vi "ArdnoManualControl.vi"() -> ()   [LabVIEW 2018, in "Arduino.lvlib"]
uses:
  Arduino.lvlib
  <vilib>/MakerHub/LINX/Public/Peripherals/Digital/Digital Write N Chans.vi
  <vilib>/MakerHub/LINX/Private/Local IO/LinxDigitalWrite.vi
  <vilib>/MakerHub/LINX/Public/Utilities/Check Channel.vi
  <vilib>/MakerHub/LINX/Public/Utilities/Open Serial.vi
  <vilib>/MakerHub/LINX/Private/Utilties/Generate Error.vi
  <vilib>/MakerHub/LINX/LMH-LINX.lvlib
panel:
  in  "Valve (A1-C8),\n comma separated":string
  in  "stop":bool
  in  "Change State\n (XOR)":bool
  in  "Period on (=Period off) (ms)":i32
  in  "All close":bool=TRUE
  in  "All open":bool
  in  "Valve (A1-C8),\n comma separated 2":string
  in  "Valve Port (Arduino)":refnum<visa-resource-name>="COM7"
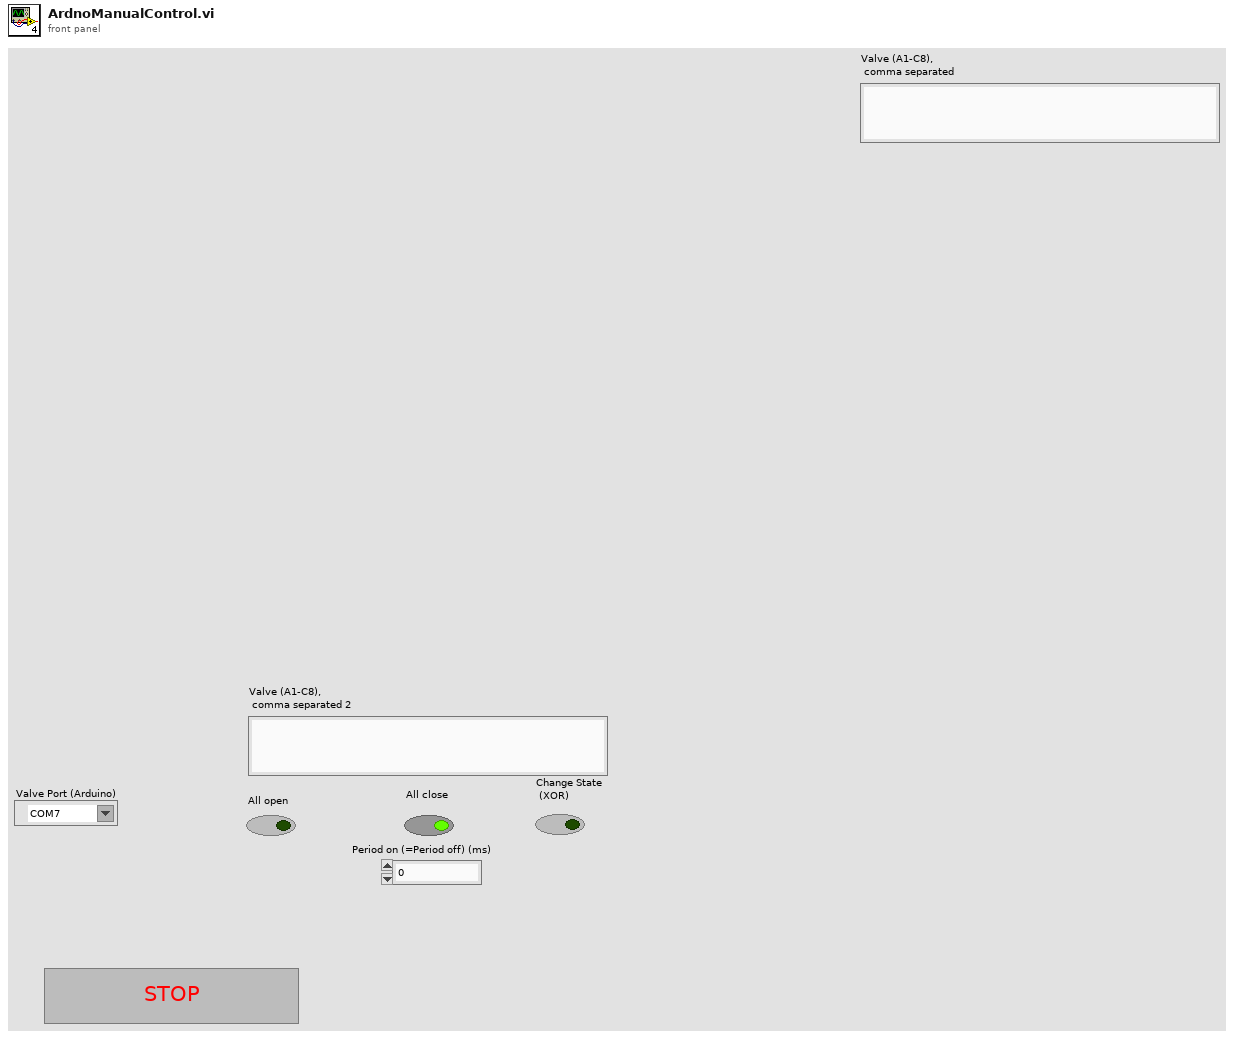
[diagram p1: front panel]
types:
  T1 = typedef "LMH-LINX.lvlib/LINX Ref.ctl" = cluster{"IO":T2, "Interface":T3, "LINX Device Config":T4}
  T2 = typedef "LMH-LINX.lvlib/Platform.ctl" = enum16{"Remote", "Local"}
  T3 = typedef "LMH-LINX.lvlib/Interface.ctl" = enum16{"Serial", "TCP"}
  T4 = typedef "LMH-LINX.lvlib/Device.lvlib/LINX Device Config.ctl" = cluster{"Interface":T3, "COM Port":refnum<visa-resource-name>, "TCP Configuration":T5, "Device Family":u8, "Device ID":u8, "Device Name":string, "TCP Ref":refnum<k5>, "Channels":T6}
  T5 = typedef "LMH-LINX.lvlib/Device.lvlib/TCP Config.ctl" = cluster{"IP Address":string, "Port":u16}
  T6 = typedef "LMH-LINX.lvlib/Channels.ctl" = cluster{"DI":u8[], "DO":u8[], "AI":u8[], "AO":u8[], "PWM":u8[], "QE":u8[], "UART":u8[], "I2C 2":u8[], "SPI":u8[], "CAN":u8[], "Servo":u8[], "AI Ref (V)":dbl, "AI Resolution (Bits)":u8, "AO Ref (V)":dbl, "AO Resolution (Bits)":u8}
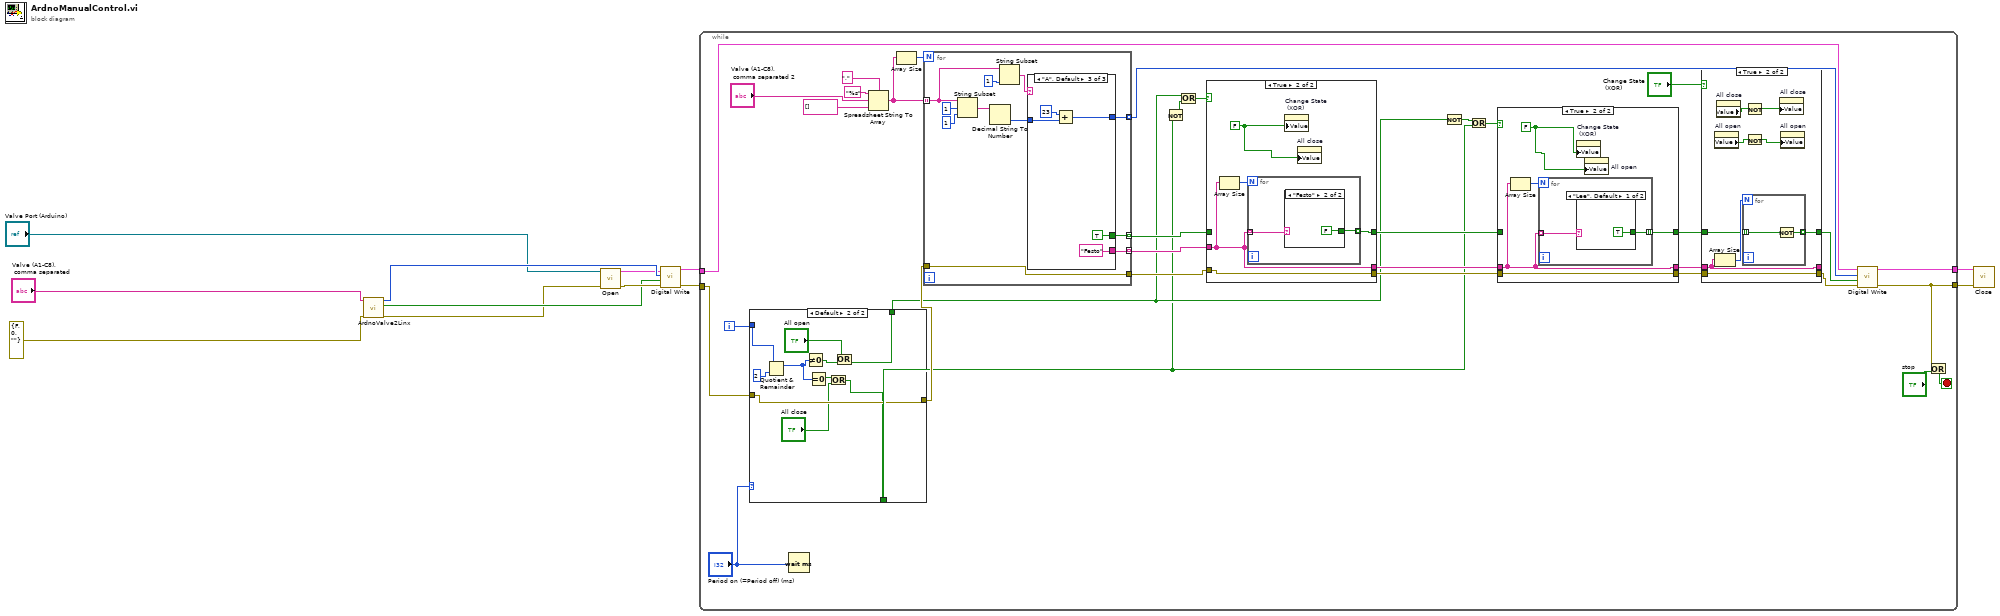
[diagram p0: block diagram]
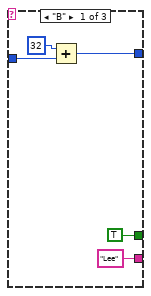
[diagram p2: hidden frame]
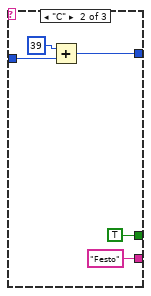
[diagram p3: hidden frame]
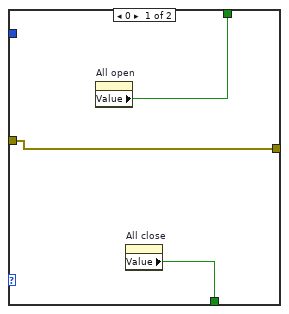
[diagram p4: hidden frame]
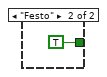
[diagram p7: hidden frame]
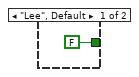
[diagram p9: hidden frame]
diagram:
  n1 = call "ArdnoValve2Linx.vi"("error in (no error)"=errorcluster {"status"=FALSE, "code"=0, "source"=""}, "Valve (A1-C8),\n comma separated"="Valve (A1-C8),\n comma separated") -> ("error out"=w5:errorcluster, "Closed State"=w6:bool[], "Linx Port"=w7:i32[])  [unwired: 7 in]
  n2 = call-poly <vilib>:"Open.vi"("Error In"=w5, "Serial Port"="Valve Port (Arduino)") -> ("Error Out"=w10:errorcluster, "LINX Resource"=w1:T1)  [unwired: 7 in, 1 out]
  n3 = call-poly <vilib>:"Digital Write.vi"("Error In"=w10, "Values"=w6, "DO Channels"=w7, "LINX Resource"=w1) -> ("Error Out"=w9:errorcluster, "LINX Resource"=w8:T1)  [unwired: 6 in]
  n4 = while {
    tunnel: w8 -> [w37]
    tunnel: w9 -> [w26]
    tunnel: [w35] -> w11
    tunnel: [w36] -> w12
    i -> [w28]
    stop <- w34 stop-if-true
    n5 = case shown="Default" "Period on (=Period off) (ms)" {
      tunnel: w28 -> [_ w85]
      tunnel: w26 -> [w75 w82]
      tunnel: [w75 w82] -> w24
      tunnel: [w74 w77] -> w20
      tunnel: [w73 w80] -> w19
      frame 0 {
        n6 = property on="All open" class="Bool (strict)"() -> ("Value"=w74:bool)  [unwired: 2 in, 2 out]
        n7 = property on="All close" class="Bool (strict)"() -> ("Value"=w73:bool)  [unwired: 2 in, 2 out]
      }
      frame Default {
        n8 = Quotient & Remainder(x=w85, y=2) -> (x-y*floor(x/y)=w83:i32)  [unwired: 1 out]
        n9 = Not Equal To 0?(x=w83) -> (x != 0?=w81:bool)
        n10 = Equal To 0?(x=w83) -> (x = 0?=w79:bool)
        n11 = Or(x=w79, y="All close") -> (x .or. y?=w80:bool)
        n12 = Or(x="All open", y=w81) -> (x .or. y?=w77:bool)
      }
    }
    n13 = Wait (ms)(milliseconds to wait="Period on (=Period off) (ms)") -> ()  [unwired: 1 out]
    n14 = Spreadsheet String To Array(delimiter (Tab)=",", format string="%s", spreadsheet string="Valve (A1-C8),\n comma separated 2", array type (2D Dbl)=string[] []) -> (array=w18:string[])
    n15 = Array Size(array=w18) -> (size(s)=w17:i32)
    n16 = for {
      N: w17 -> [_]
      tunnel: w18 -> [w54] mode=indexing
      tunnel: [w49] -> w45 mode=indexing
      tunnel: [w50] -> w46 mode=indexing
      tunnel: [w48] -> w38 mode=indexing
      tunnel: [w47] -> w25
      tunnel: w24 -> [w47]
      n17 = String Subset(string=w54, offset (0)=1, length (rest)=1 ("length (rest)")) -> (substring=w52:string)
      n18 = Decimal String To Number(string=w52) -> (number=w51:i32)  [unwired: 2 in, 1 out]
      n19 = String Subset(string=w54, length (rest)=1 ("length (rest)")) -> (substring=w56:string)  [unwired: 1 in]
      n20 = case shown="\"A\", Default" w56 {
        tunnel: [w61 w66 w71] -> w48
        tunnel: w51 -> [w60 w65 w70]
        tunnel: ["Lee" "Festo" "Festo"] -> w50
        tunnel: [TRUE TRUE TRUE] -> w49
        frame "B" {
          n21 = Add(x=32, y=w60) -> (x+y=w61:i32)
        }
        frame "C" {
          n22 = Add(x=39, y=w65) -> (x+y=w66:i32)
        }
        frame "A", Default {
          n23 = Add(x=23, y=w70) -> (x+y=w71:i32)
        }
      }
    }
    n24 = Not(x=w19) -> (.not. x?=w29:bool)
    n25 = Or(x=w20, y=w29) -> (x .or. y?=w30:bool)
    n26 = case shown="True" w30 {
      tunnel: w46 -> [w110 w114]
      tunnel: w45 -> [w111 _]
      tunnel: [w111 w115] -> w44
      tunnel: [w110 w114] -> w43
      tunnel: w25 -> [_ w112]
      tunnel: [_ w112] -> w23
      frame False {
      }
      frame True {
        w113 = FALSE
        n27 = Array Size(array=w114) -> (size(s)=w116:i32)
        n28 = for {
          N: w116 -> [_]
          tunnel: w114 -> [w118] mode=indexing
          tunnel: [w117] -> w115 mode=indexing
          n29 = case shown="\"Festo\"" w118 {
            tunnel: [FALSE FALSE] -> w117
            frame "Lee", Default {
            }
            frame "Festo" {
            }
          }
        }
        n30 = property on="Change State\n (XOR)" class="Bool (strict)"("Value"=w113) -> ()  [unwired: 2 in, 2 out]
        n31 = property on="All close" class="Bool (strict)"("Value"=w113) -> ()  [unwired: 2 in, 2 out]
      }
    }
    n32 = Not(x=w20) -> (.not. x?=w31:bool)
    n33 = Or(x=w31, y=w19) -> (x .or. y?=w32:bool)
    n34 = case shown="True" w32 {
      tunnel: w43 -> [w99 w103]
      tunnel: w44 -> [w100 _]
      tunnel: [w100 w104] -> w41
      tunnel: [w99 w103] -> w40
      tunnel: w23 -> [_ w101]
      tunnel: [_ w101] -> w22
      frame False {
      }
      frame True {
        w102 = FALSE
        n35 = Array Size(array=w103) -> (size(s)=w105:i32)
        n36 = for {
          N: w105 -> [_]
          tunnel: w103 -> [w107] mode=indexing
          tunnel: [w106] -> w104 mode=indexing
          n37 = case shown="\"Lee\", Default" w107 {
            tunnel: [TRUE TRUE] -> w106
            frame "Lee", Default {
            }
            frame "Festo" {
            }
          }
        }
        n38 = property on="Change State\n (XOR)" class="Bool (strict)"("Value"=w102) -> ()  [unwired: 2 in, 2 out]
        n39 = property on="All open" class="Bool (strict)"("Value"=w102) -> ()  [unwired: 2 in, 2 out]
      }
    }
    n40 = case shown="True" "Change State\n (XOR)" {
      tunnel: w40 -> [w86 w94]
      tunnel: w41 -> [w87 w93]
      tunnel: [w87 w95] -> w39
      tunnel: [w86 w94] -> _
      tunnel: w22 -> [_ w92]
      tunnel: [_ w92] -> w21
      frame False {
      }
      frame True {
        n41 = property on="All open" class="Bool (strict)"() -> ("Value"=w88:bool)  [unwired: 2 in, 2 out]
        n42 = Array Size(array=w94) -> (size(s)=w96:i32)
        n43 = property on="All close" class="Bool (strict)"() -> ("Value"=w91:bool)  [unwired: 2 in, 2 out]
        n44 = for {
          N: w96 -> [_]
          tunnel: [w97] -> w95 mode=indexing
          tunnel: w93 -> [w98] mode=indexing
          n45 = Not(x=w98) -> (.not. x?=w97:bool)
        }
        n46 = Not(x=w91) -> (.not. x?=w90:bool)
        n47 = Not(x=w88) -> (.not. x?=w89:bool)
        n48 = property on="All close" class="Bool (strict)"("Value"=w90) -> ()  [unwired: 2 in, 2 out]
        n49 = property on="All open" class="Bool (strict)"("Value"=w89) -> ()  [unwired: 2 in, 2 out]
      }
    }
    n50 = call-poly <vilib>:"Digital Write.vi"("Error In"=w21, "Values"=w39, "DO Channels"=w38, "LINX Resource"=w37) -> ("Error Out"=w35:errorcluster, "LINX Resource"=w36:T1)  [unwired: 6 in]
    n51 = Or(x=w35, y="stop") -> (x .or. y?=w34:bool)
  }
  n52 = call <vilib>:"Close.vi"("Error In"=w11, "LINX Resource"=w12) -> ()  [unwired: 9 in, 1 out]
